vi "Begin Transaction.vi"(8 "error in (no error)":errorcluster, 11 "DbConnection in":refnum<class "DbConnection.lvclass">) -> (0 "error out":errorcluster, 3 "DbConnection out":refnum<class "DbConnection.lvclass">)   [LabVIEW 2020, in "ORM.lvlib" / "DbConnection.lvclass"]
uses:
  DbConnection.lvclass
  DbConnection.lvclass/DbConnection.ctl
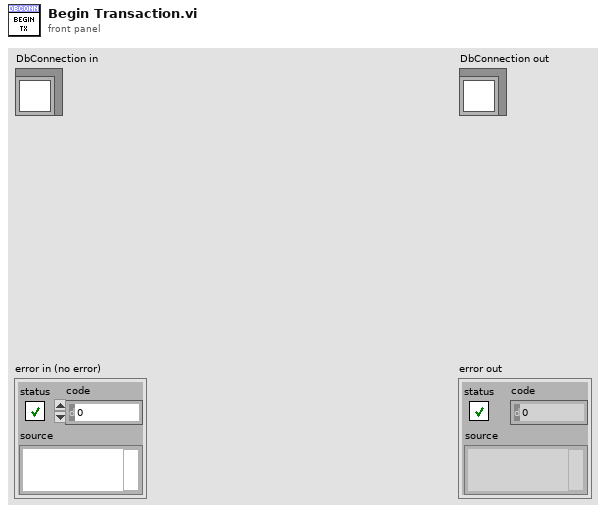
[diagram p1: front panel]
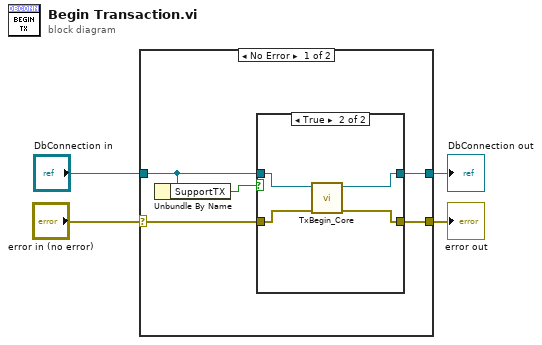
[diagram p0: block diagram]
diagram:
  n1 = case shown="No Error" "error in (no error)" {
    selector: "error in (no error)" -> [w8 w17]
    tunnel: [w7 w17] -> w3
    tunnel: [w9 w16] -> w1
    tunnel: "DbConnection in" -> [w6 w16]
    frame No Error {
      n2 = Unbundle By Name(w6) -> ("SupportTX"=w5:bool)
      n3 = case shown="True" w5 {
        tunnel: w6 -> [w11 w14]
        tunnel: [w11 w12] -> w9
        tunnel: w8 -> [w10 w15]
        tunnel: [w10 w13] -> w7
        frame False {
        }
        frame True {
          n4 = call-dynamic "TxBegin_Core.vi"("error in (no error)"=w15, "DbConnection in"=w14) -> ("error out"=w13:errorcluster, "DbConnection out"=w12:refnum<class "DbConnection.lvclass">)  [unwired: 8 in]
        }
      }
    }
    frame Error {
    }
  }
  "error out" <- w3
  "DbConnection out" <- w1
